vi "while loop count.vi"() -> ()   [LabVIEW 2016]
panel:
  out "Loop Count":i32
  in  "Power":bool
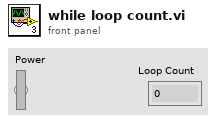
[diagram p1: front panel]
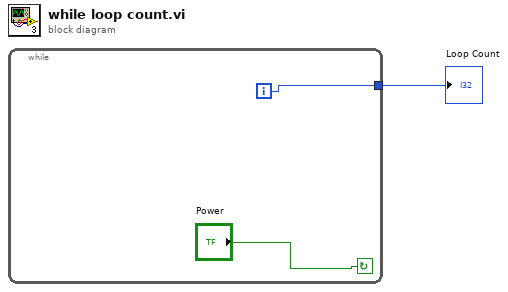
[diagram p0: block diagram]
diagram:
  n1 = while {
    tunnel: [w3] -> w1
    i -> [w3]
    stop <- "Power" continue-if-true
  }
  "Loop Count" <- w1
